vi "turn_off_indicators.vi"(8 "error in (no error)":errorcluster, 9 "Message Queues in":T1, 11 "test mode in":T2(ring)) -> (0 "error out":errorcluster, 1 "Message Queues out":T1, 3 "test mode out":T2(ring))   [LabVIEW 2015]
uses:
  support/Message Queue/All Message Queues.ctl
  support/Message Queue/Message Cluster.ctl
  support/Message Queue/Enqueue Message (Single).vi
  support/Message Queue/Message Queue.lvlib
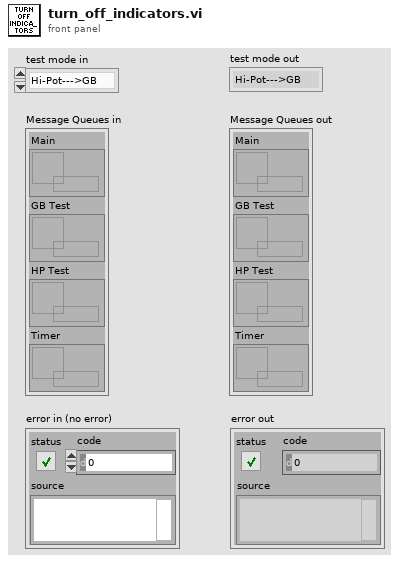
[diagram p1: front panel]
types:
  T1 = typedef "Message Queue.lvlib/All Message Queues.ctl" = cluster{"Main":refnum<queue>, "GB Test":refnum<queue>, "HP Test":refnum<queue>, "Timer":refnum<queue>}
  T2 = enum16{"Hi-Pot--->GB", "GB--->Hi-Pot", "Hi-Pot only", "GB only"}
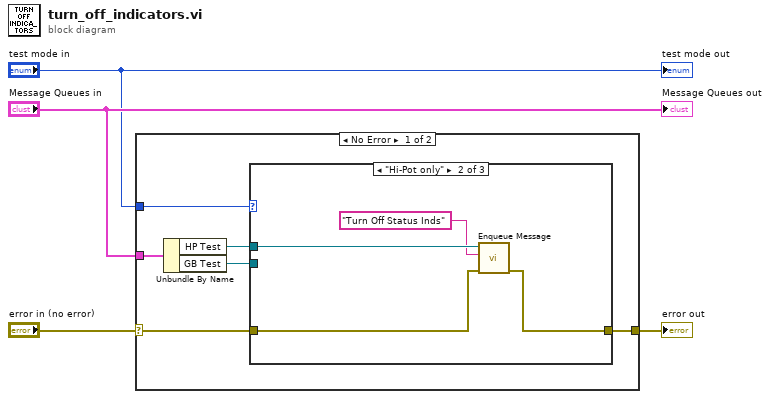
[diagram p0: block diagram]
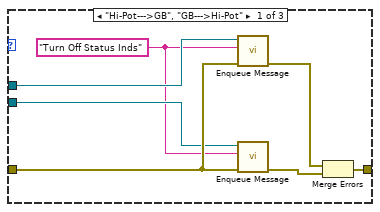
[diagram p2: hidden frame]
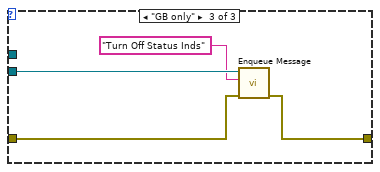
[diagram p3: hidden frame]
diagram:
  n1 = case shown="No Error" "error in (no error)" {
    selector: "error in (no error)" -> [w6 w26]
    tunnel: "Message Queues in" -> [w10 _]
    tunnel: "test mode in" -> [w9 _]
    tunnel: [w5 w26] -> w2
    frame No Error {
      n2 = Unbundle By Name(w10) -> ("HP Test"=w8:refnum<queue>, "GB Test"=w7:refnum<queue>)
      n3 = case shown="\"Hi-Pot only\"" w9 {
        tunnel: w8 -> [w16 w21 _]
        tunnel: w7 -> [w15 _ w25]
        tunnel: w6 -> [w17 w19 w24]
        tunnel: [w12 w18 w23] -> w5
        frame "Hi-Pot--->GB", "GB--->Hi-Pot" {
          w11 = "Turn Off Status Inds"
          n4 = call-poly "Enqueue Message.vi"("error in (no error)"=w17, "Message"=w11, "Message Queue"=w16) -> ("error out"=w14:errorcluster)  [unwired: 7 in, 1 out]
          n5 = call-poly "Enqueue Message.vi"("error in (no error)"=w17, "Message"=w11, "Message Queue"=w15) -> ("error out"=w13:errorcluster)  [unwired: 7 in, 1 out]
          n6 = Merge Errors(w14, w13) -> (w12:errorcluster)
        }
        frame "Hi-Pot only" {
          n7 = call-poly "Enqueue Message.vi"("error in (no error)"=w19, "Message"="Turn Off Status Inds", "Message Queue"=w21) -> ("error out"=w18:errorcluster)  [unwired: 7 in, 1 out]
        }
        frame "GB only" {
          n8 = call-poly "Enqueue Message.vi"("error in (no error)"=w24, "Message"="Turn Off Status Inds", "Message Queue"=w25) -> ("error out"=w23:errorcluster)  [unwired: 7 in, 1 out]
        }
      }
    }
    frame Error {
    }
  }
  "error out" <- w2
  "test mode out" <- "test mode in"
  "Message Queues out" <- "Message Queues in"
